vi "cno_scale.vi"(0 "P":dbl[](array[numeric]), 1 "cno data":T1, 5 "L":dbl[](array[numeric]), 9 "H":dbl[][](array[numeric]), 11 "OB":dbl[](array[numeric]), 12 "PB":dbl[][](array[numeric])) -> (2 "cno data":T1, 4 "P":dbl[](array[numeric]), 6 "L":dbl[](array[numeric]), 8 "SCALE":dbl[](array[numeric]), 10 "H":dbl[][](array[numeric]), 14 "PB":dbl[][](array[numeric]), 15 "OB":dbl[](array[numeric]))   [LabVIEW 2020, in "NI_Gmath.lvlib"]
uses:
  <vilib>/gmath/NI_Gmath.lvlib
  <vilib>/gmath/NumericalOptimization/cno_data.ctl
  <vilib>/Analysis/baseanly.llb/Real Outer Product.vi
  <vilib>/Analysis/Matrix/Numeric/Conversions/Matrix To Array - RM.vi
  <vilib>/Analysis/NI_AALBase.lvlib
  <vilib>/Analysis/Matrix/NI_Matrix.lvlib
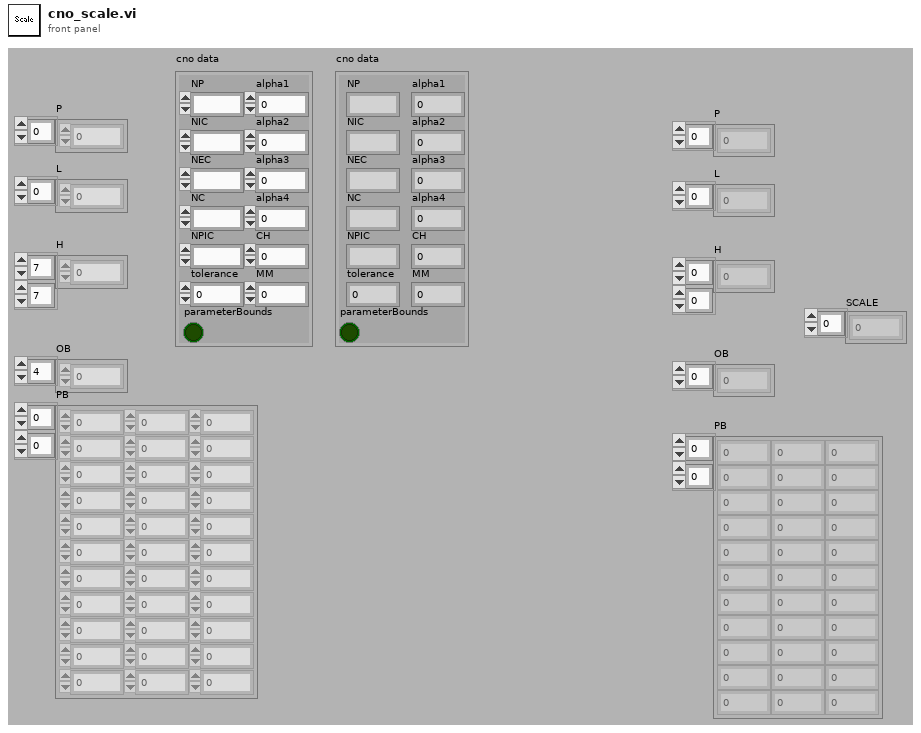
[diagram p1: front panel]
types:
  T1 = typedef "NI_Gmath.lvlib/cno_data.ctl" = cluster{"NP":i32, "NIC":i32, "NEC":i32, "NC":i32, "NPIC":i32, "parameterBounds":bool, "alpha1":dbl, "alpha2":dbl, "alpha3":dbl, "alpha4":dbl, "CH":i32, "MM":i32, "tolerance":dbl}
  T2 = typedef "NI_Matrix.lvlib/RealMatrix.ctl" = dbl[][]
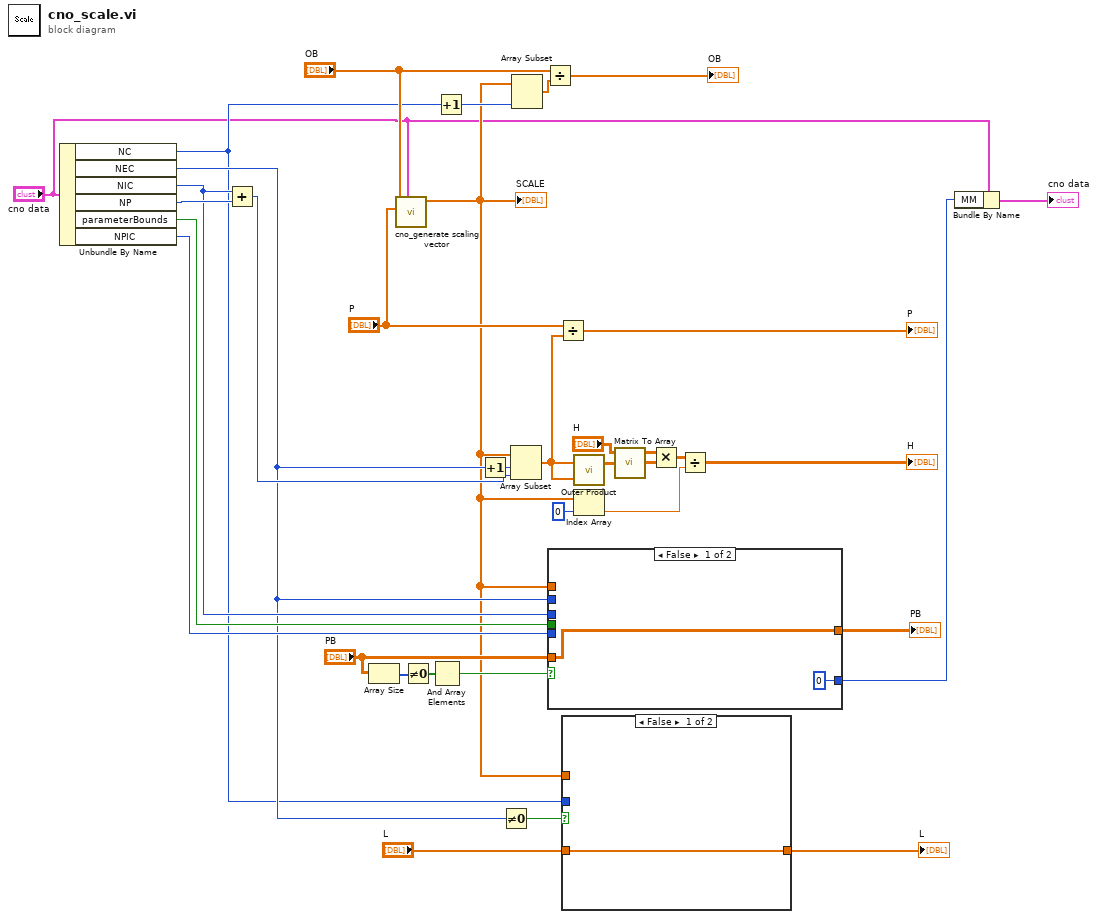
[diagram p0: block diagram]
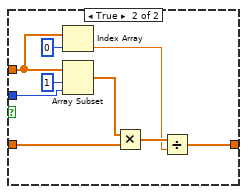
[diagram p2: hidden frame]
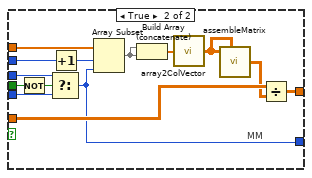
[diagram p3: hidden frame]
diagram:
  n1 = Unbundle By Name("cno data") -> ("NC"=w15:i32, "NEC"=w16:i32, "NIC"=w20:i32, "NP"=w29:i32, "parameterBounds"=w21:bool, "NPIC"=w19:i32)
  n2 = Add(x=w20, y=w29) -> (x+y=w30:i32)
  n3 = Array Size(array="PB") -> (size(s)=w25:i32[])
  n4 = call <vilib>:"cno_generate scaling vector.vi"("cno data"="cno data", "P"="P", "OB"="OB") -> ("scaling vector"=w6:dbl[])  [unwired: 8 in]
  "SCALE" <- w6
  n5 = Not Equal To 0?(x=w25) -> (x != 0?=w24:bool[])
  n6 = And Array Elements(Boolean array=w24) -> (logical AND=w23:bool)
  n7 = Increment(x=w15) -> (x+1=w34:i32)
  n8 = Increment(x=w16) -> (x+1=w31:i32)
  n9 = Not Equal To 0?(x=w16) -> (x != 0?=w17:bool)
  n10 = Array Subset(array=w6, index=w31, length=w30) -> (w12:dbl[])
  n11 = Array Subset(array=w6, length=w34) -> (w32:dbl[])  [unwired: 1 in]
  n12 = Divide(x="OB", y=w32) -> (x/y=→"OB":dbl[])
  n13 = case shown="False" w23 {
    tunnel: "PB" -> [w36 w42]
    tunnel: w21 -> [_ w50]
    tunnel: w20 -> [_ w48]
    tunnel: w19 -> [_ w47]
    tunnel: w16 -> [_ w46]
    tunnel: w6 -> [_ w45]
    tunnel: [w36 w38] -> w18
    tunnel: [0 w37] -> w4
    frame False {
    }
    frame True {
      # "MM"
      n14 = Not(x=w50) -> (.not. x?=w49:bool)
      n15 = Select(t=w48, s=w49, f=w47) -> (s? t:f=w37:i32)
      n16 = Increment(x=w46) -> (x+1=w44:i32)
      n17 = Array Subset(array=w45, index=w44, length=w37) -> (w43:dbl[])
      n18 = Build Array (concatenate)(w43, w43) -> (w41:dbl[])
      n19 = call <vilib>:"array2ColVector.vi"("vector"=w41) -> ("col vector"=w40:dbl[][])
      n20 = call <vilib>:"assembleMatrix.vi"("A"=w40, "B"=w40) -> ("ABCD"=w39:dbl[][])  [unwired: 3 in]
      n21 = Divide(x=w42, y=w39) -> (x/y=w38:dbl[][])
    }
  }
  "PB" <- w18
  n22 = Divide(x="P", y=w12) -> (x/y=→"P":dbl[])
  n23 = case shown="False" w17 {
    tunnel: w6 -> [_ w56]
    tunnel: w15 -> [_ w59]
    tunnel: "L" -> [w51 w58]
    tunnel: [w51 w52] -> w13
    frame False {
    }
    frame True {
      n24 = Index Array(array=w56, index=0) -> (element=w53:dbl)
      n25 = Array Subset(array=w56, index=1, length=w59) -> (w57:dbl[])
      n26 = Multiply(x=w57, y=w58) -> (x*y=w54:dbl[])
      n27 = Divide(x=w54, y=w53) -> (x/y=w52:dbl[])
    }
  }
  "L" <- w13
  n28 = call-poly <vilib>:"Outer Product.vi"("Y Vector"=w12, "X Vector"=w12) -> ("Outer Product"=w1:T2)  [unwired: 1 out]
  n29 = Index Array(array=w6, index=0) -> (element=w8:dbl)
  n30 = call-poly <vilib>:"Matrix To Array.vi"("Real Matrix"=w1) -> ("Real 2D Array"=w2:dbl[][])
  n31 = Multiply(x="H", y=w2) -> (x*y=w9:dbl[][])
  n32 = Divide(x=w9, y=w8) -> (x/y=→"H":dbl[][])
  n33 = Bundle By Name(cluster="cno data", "MM"=w4) -> (→"cno data":T1)
